vi "Status Channel Status Query.vi"(0 "VISA resource name":refnum<visa-resource-name>, 7 "Query Reg  (0:Summary Enable)":u8(slide) scale=0.0..2.0, 11 "error in (no error)":errorcluster) -> (4 "VISA resource name out":refnum<visa-resource-name>, 8 "Status Chan Reg (F:Disable)":bool[](array[boolean]), 15 "error out":errorcluster)   [LabVIEW 2015, in "Chroma ATE 6310.lvlib"]
doc: "The VI returns the setting of selected register in the Channel Status register group.\n\nThe Channel Status register offers you one or more channel status conditions,which indicate certain errors or faults have occurred on specific channel."
uses:
  <instrlib>/Chroma ATE 6310/Chroma ATE 6310.lvlib
panel:
  # "OC                OV                 OP                 RV                OT"
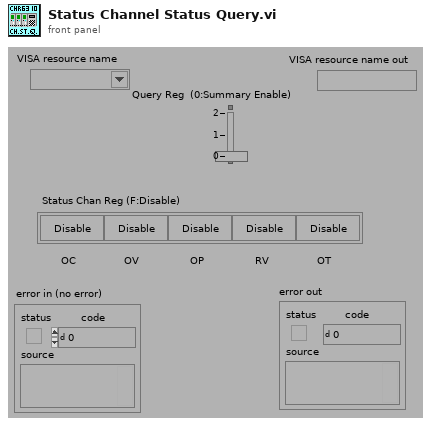
[diagram p1: front panel]
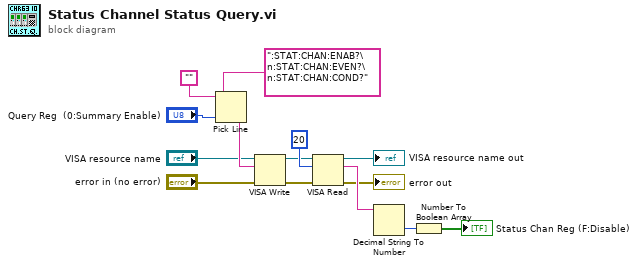
[diagram p0: block diagram]
diagram:
  n1 = Pick Line(string ("")="", multi-line string=":STAT:CHAN:ENAB?\n:STAT:CHAN:EVEN?\n:STAT:CHAN:COND?", line index="Query Reg  (0:Summary Enable)") -> (output string=w8:string)
  n2 = VISA Write(VISA resource name="VISA resource name", write buffer=w8, error in (no error)="error in (no error)") -> (VISA resource name out=w11:refnum<visa-resource-name>, error out=w10:errorcluster)  [unwired: 1 out]
  n3 = VISA Read(VISA resource name=w11, byte count=u32 20, error in (no error)=w10) -> (VISA resource name out=→"VISA resource name out":refnum<visa-resource-name>, read buffer=w13:string, error out=→"error out":errorcluster)  [unwired: 1 out]
  n4 = Decimal String To Number(string=w13) -> (number=w14:i32)  [unwired: 2 in, 1 out]
  n5 = Number To Boolean Array(number=w14) -> (Boolean array=→"Status Chan Reg (F:Disable)":bool[])
